vi "Actor Core.vi"(8 "error in":cluster{"状态":bool, "代码":i32, "源":string} caption="错误输入", 11 "MapDisplayer":refnum<class "Map.lvclass">) -> (0 "error out":cluster{"状态":bool, "代码":i32, "源":string} caption="错误输出", 3 "操作者输出":refnum<class "Actor.lvclass">)   [LabVIEW 2014, in "Map.lvlib" / "Map.lvclass"]
doc: "Actor Core.vi包含操作者的主要消息处理循环。操作者通常位于该循环中，在各种消息到达时对消息进行处理。如Do.vi消息返回任何错误，该循环将停止运行，错误代码43将被作为“无错误停止”的标准信号发送给调用方。如需更改上述行为，可在子孙类的Handle Error.vi中对该部分逻辑进行重写。"
uses:
  Map.lvclass
  <vilib>/ActorFramework/Actor/Actor.lvclass
  MapBuilder/Robot_Position.ctl
  <vilib>/ActorFramework/Actor/Actor.lvclass/Actor.ctl
  Map.lvclass/Map.ctl
  Wrapper_lib/zsActor/ActorWrapper.lvclass
panel:
  out "robot position":T1
  out "平面俯视图":T2(plugin-control)
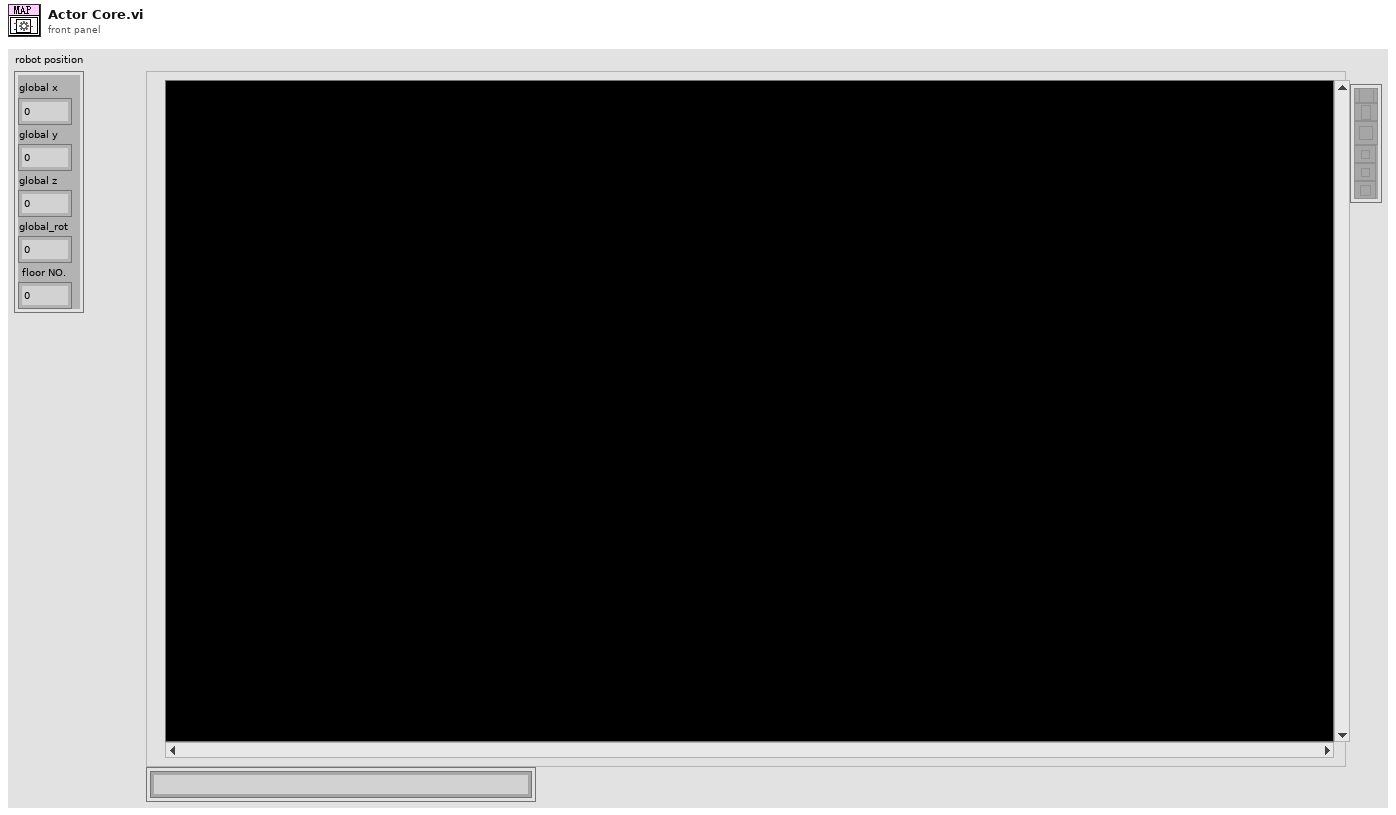
[diagram p1: front panel]
types:
  T1 = typedef "Robot_Position.ctl" = cluster{"global x":dbl, "global y":dbl, "global z":dbl, "global_rot":dbl, " floor NO.":dbl}
  T2 = typedef "IMAQ Image.ctl" = refnum<image>
  T3 = typedef "NI_Matrix.lvlib/RealMatrix.ctl" = dbl[][]
  T4 = cluster{"District Name":string, "Alias":string, "District Type":string, "Floor NO.":string, "Data Matrix":T3, "Path array":string[], "Path Coodinate":T3}[]
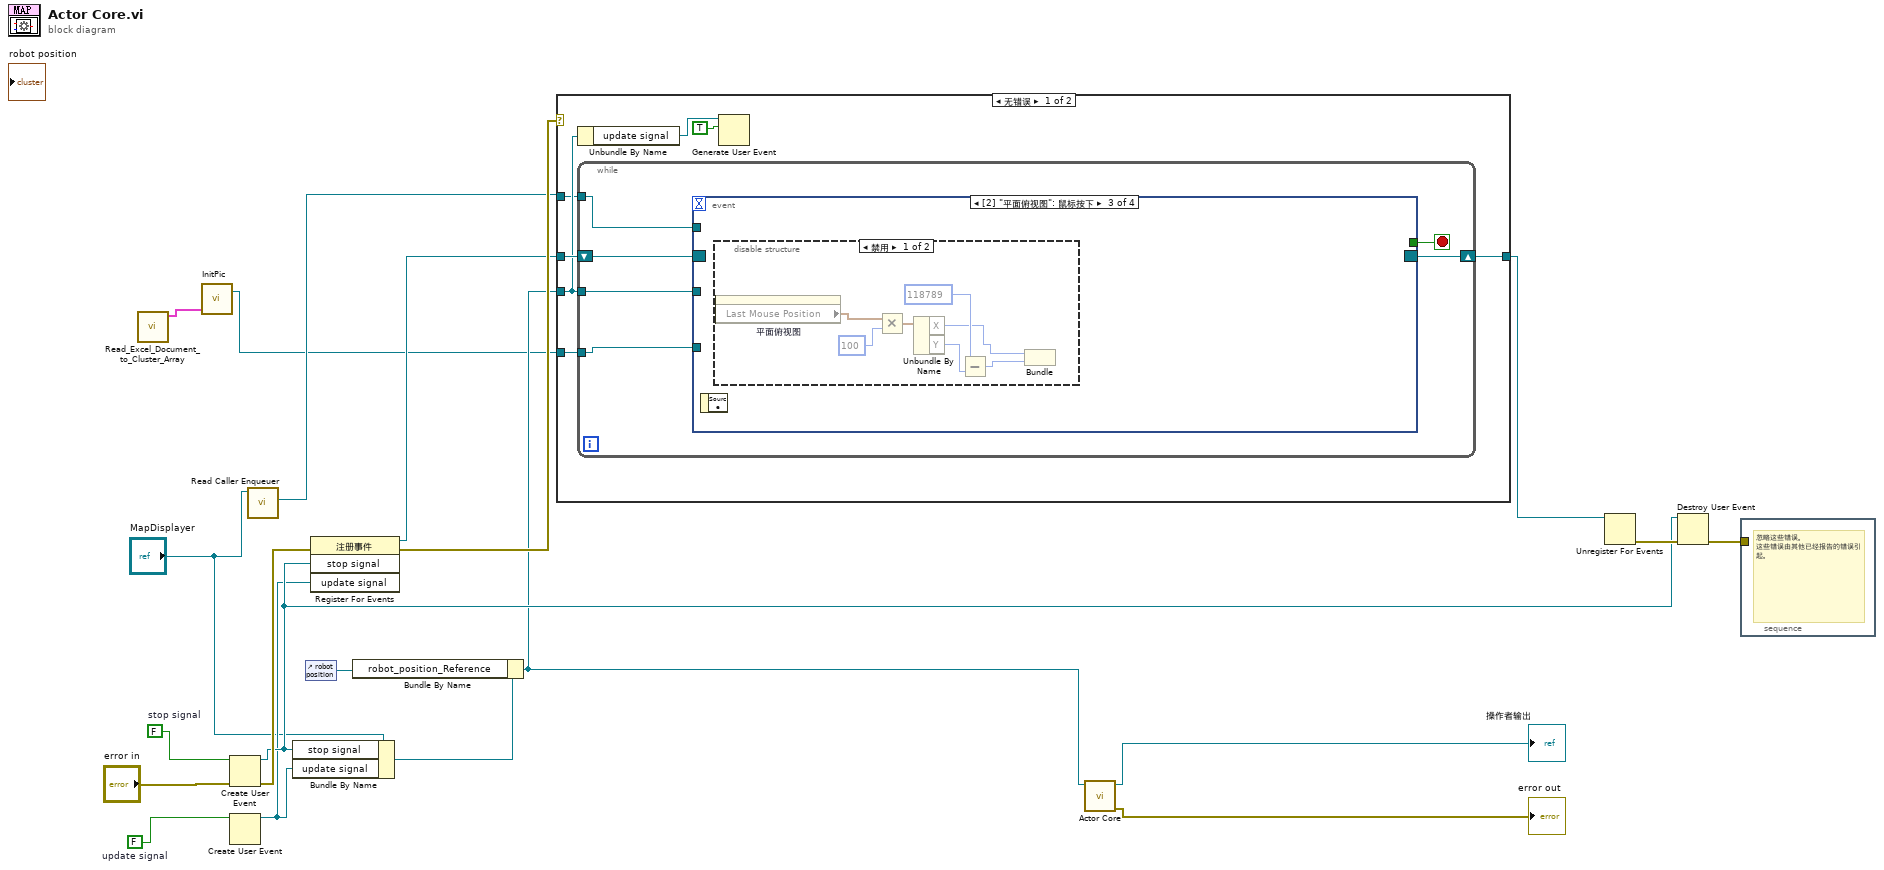
[diagram p0: block diagram]
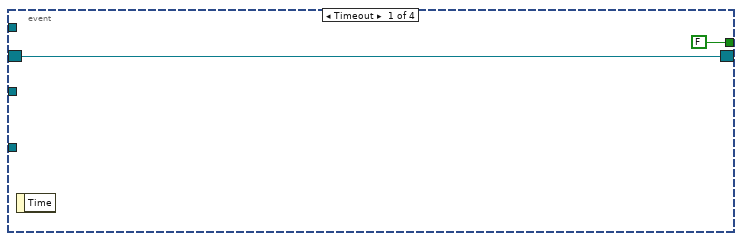
[diagram p2: hidden frame]
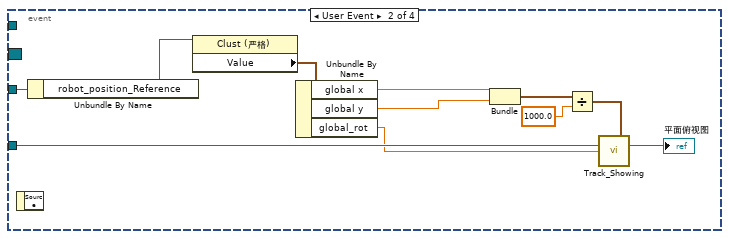
[diagram p3: hidden frame]
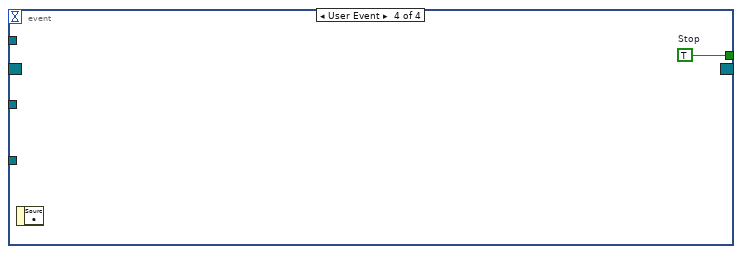
[diagram p5: hidden frame]
diagram:
  w7 = FALSE  # update signal
  w15 = FALSE  # stop signal
  n1 = call "Read_Excel_Document_to_Cluster_Array.vi"() -> ("Cluster of 7 Type Data_4F"=w3:T4)  [unwired: 8 in, 3 out]
  n2 = call "InitPic.vi"("Cluster of 7 Type Data"=w3) -> ("Image Out 2"=w2:T2)  [unwired: 3 in]
  n3 = Create User Event(user event datatype=w15, error in="error in") -> (user event=w9:refnum<user-event>, error out=w16:errorcluster)
  n4 = Create User Event(user event datatype=w7) -> (user event=w6:refnum<user-event>)  [unwired: 1 in, 1 out]
  n5 = call <vilib>:"Read Caller Enqueuer.vi"("Actor"="MapDisplayer") -> ("Caller Enqueuer"=w4:refnum<class "Message Enqueuer.lvclass">)  [unwired: 10 in]
  n6 = Bundle By Name(cluster="MapDisplayer", "stop signal"=w9, "update signal"=w6) -> (w17:refnum<class "Map.lvclass">)
  n7 = control-ref of="robot position"() -> (w1:refnum<vi>)
  n8 = register-events(error in=w16, w9, w6) -> (reference out=w13:refnum<event-registration>, error out=w14:errorcluster)  [unwired: 1 in]
  n9 = Bundle By Name(cluster=w17, "robot_position_Reference"=w1) -> (w8:refnum<class "Map.lvclass">)
  n10 = case shown="无错误" w14 {
    tunnel: w13 -> [w27 w55]
    tunnel: [w26 w55] -> w12
    tunnel: w8 -> [w25 _]
    tunnel: w4 -> [w22 _]
    tunnel: w2 -> [w21 _]
    frame No Error {
      n11 = Unbundle By Name(w25) -> ("update signal"=w24:refnum<user-event>)
      n12 = while {
        shift-right: [w32] -> w26
        shift-left: w27 -> [w33]
        tunnel: w25 -> [w30]
        tunnel: w22 -> [w29]
        tunnel: w21 -> [w28]
        stop <- w31 stop-if-true
        n13 = event shown="[2] \"平面俯视图\": 鼠标按下" {
          selector: w33 -> [w35 _ _ _]
          dyn-events: [w35 _ _ _] -> w32
          timeout: _ -> [_ _ _ _]
          tunnel: [FALSE ("Stop") _ _ w54] -> w31
          tunnel: w30 -> [_ w44 _ _]
          tunnel: w29 -> [_ _ _ _]
          tunnel: w28 -> [_ w39 _ _]
          event Timeout {
            n14 = event-data() -> ()  [unwired: 1 in, 1 out]
          }
          event User Event {
            n15 = event-data() -> ()  [unwired: 1 in, 1 out]
            n16 = Unbundle By Name(w44) -> ("robot_position_Reference"=w45:refnum<vi>)
            n17 = property class="Clust (严格)"(reference=w45) -> ("Value"=w46:T1)  [unwired: 1 in, 2 out]
            n18 = Unbundle By Name(w46) -> ("global x"=w40:dbl, "global y"=w37:dbl, "global_rot"=w36:dbl)
            n19 = Bundle("global x"=w40, "global y"=w37) -> (w43:cluster{"global x":dbl, "global y":dbl})  [unwired: 1 in]
            n20 = Divide(x=w43, y=1000.0) -> (x/y=w41:cluster{"global x":dbl, "global y":dbl})
            n21 = call "Track_Showing.vi"("NewNodeM"=w41, "Image In 2"=w39, "数值"=w36) -> ("Image Out 2"=→"平面俯视图":T2)  [unwired: 12 in]
          }
          event "平面俯视图": Mouse Down {
            n22 = event-data() -> ()  [unwired: 1 in, 1 out]
            n23 = disable-structure shown="禁用" {
              frame Disabled {
                n24 = property on="平面俯视图" class="ImageControl"() -> ("Last Mouse Position"=w53:cluster{"X":i32, "Y":i32})  [unwired: 2 in, 2 out]
                n25 = Multiply(x=w53, y=100) -> (x*y=w51:cluster{"X":i32, "Y":i32})
                n26 = Unbundle By Name(w51) -> ("X"=w48:i32, "Y"=w50:i32)
                n27 = Subtract(x=118789, y=w50) -> (x-y=w47:i32)
                n28 = Bundle("X"=w48, w47) -> ()  [unwired: 1 in, 1 out]
              }
              frame Enabled {
              }
            }
          }
          event User Event {
            w54 = TRUE  # Stop
            n29 = event-data() -> ()  [unwired: 1 in, 1 out]
          }
        }
      }
      n30 = Generate User Event(user event=w24, event data cluster=TRUE ("事件数据")) -> ()  [unwired: 2 in, 2 out]
    }
    frame Error {
    }
  }
  n31 = call-parent "Actor Core.vi"("Actor in"=w8) -> ("error out"=→"error out":errorcluster, "Actor out"=→"操作者输出":refnum<class "Actor.lvclass">)  [unwired: 9 in]
  n32 = Unregister For Events(event registration refnum=w12) -> (error out=w11:errorcluster)  [unwired: 1 in]
  n33 = Destroy User Event(user event=w9, error in=w11) -> (error out=w10:errorcluster)
  n34 = stacked-sequence {
    tunnel: w10 -> [_]
    frame #0 {
      # "忽略这些错误。\n这些错误由其他已经报告的错误引起。"
    }
  }
